vi "PRBS9 Unit Test.vi"() -> ()   [LabVIEW 2013]
doc: "This is the unit test for PRBS9. All 3 arrays on the UI should be different."
panel:
  out "Pass":bool
  out "Array 3":bool[](array[boolean])
  out "Array 2":bool[](array[boolean])
  out "Array":bool[](array[boolean])
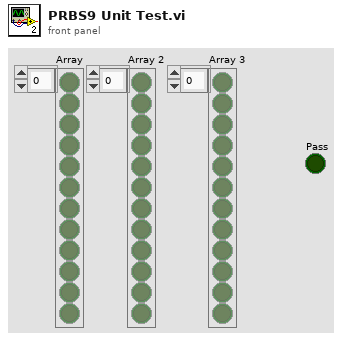
[diagram p1: front panel]
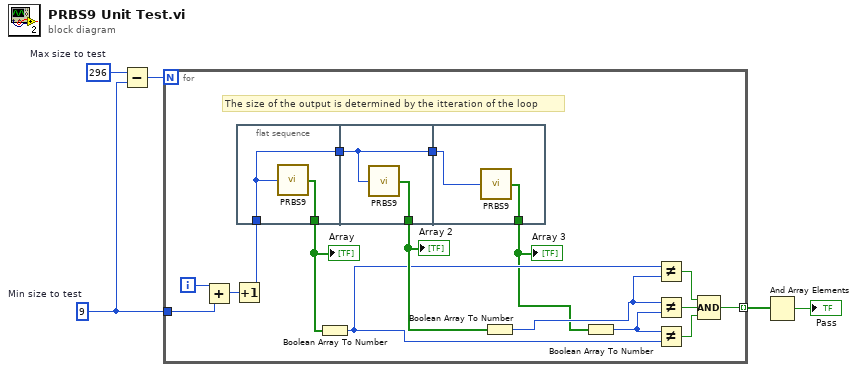
[diagram p0: block diagram]
diagram:
  w1 = 9  # Min size to test
  w3 = 296  # Max size to test
  n1 = Subtract(x=w3, y=w1) -> (x-y=w2:i32)
  n2 = for {
    N: w2 -> [_]
    tunnel: [w11] -> w5 mode=indexing
    tunnel: w1 -> [w8]
    i -> [w9]
    # "The size of the output is determined by the itteration of the loop"
    n3 = Add(x=w9, y=w8) -> (x+y=w7:i32)
    n4 = Increment(x=w7) -> (x+1=w6:i32)
    n5 = flat-sequence {
      tunnel: [w23] -> w19
      tunnel: [w22] -> w21
      tunnel: w6 -> [w22]
      tunnel: [w25] -> w18
      tunnel: [w24] -> w20
      tunnel: w21 -> [w24]
      tunnel: [w27] -> w10
      tunnel: w20 -> [w26]
      frame #0 {
        n6 = call "PRBS9.vi"("Size"=w22) -> ("Array"=w23:bool[])
      }
      frame #1 {
        n7 = call "PRBS9.vi"("Size"=w24) -> ("Array"=w25:bool[])
      }
      frame #2 {
        n8 = call "PRBS9.vi"("Size"=w26) -> ("Array"=w27:bool[])
      }
    }
    n9 = Boolean Array To Number(Boolean array=w19) -> (number=w16:u32)
    n10 = Boolean Array To Number(Boolean array=w18) -> (number=w17:u32)
    n11 = Boolean Array To Number(Boolean array=w10) -> (number=w15:u32)
    n12 = Not Equal?(x=w16, y=w17) -> (x != y?=w12:bool)
    n13 = Not Equal?(x=w17, y=w15) -> (x != y?=w13:bool)
    n14 = Not Equal?(x=w15, y=w16) -> (x != y?=w14:bool)
    n15 = Compound Arithmetic op=AND(w12, w13, w14) -> (w11:bool)
    "Array" <- w19
    "Array 2" <- w18
    "Array 3" <- w10
  }
  n16 = And Array Elements(Boolean array=w5) -> (logical AND=→"Pass":bool)
